vi "Perf Close.vi"(8 "error in (no error)":errorcluster) -> (0 "error out":errorcluster)   [LabVIEW 2017, in "Performance.lvlib"]
uses:
  Performance.lvlib
  Private FGV/Performance Methods.ctl
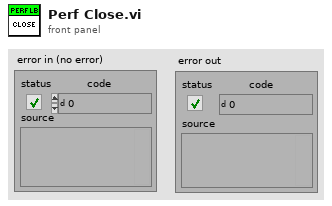
[diagram p1: front panel]
types:
  T1 = typedef "Performance.lvlib/Performance Methods.ctl" = enum16{"Init", "Get Data", "Close"}
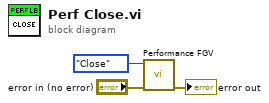
[diagram p0: block diagram]
diagram:
  n1 = call "Performance FGV.vi"("error in (no error)"="error in (no error)", "Performance Methods"=Performance_Methods."Close") -> ("error out"=→"error out":errorcluster)  [unwired: 8 in, 1 out]
